vi "Delimiter Write 1.vi"(4 "error in (no error)":errorcluster, 5 "Value":T1, 6 "Container State":T3, 7 "Display State In":T2) -> (0 "error out":errorcluster, 3 "Display State Out":T2)   [LabVIEW 2012, in "Intellisense Xcontrol.xctl"]
uses:
  Intellisense Xcontrol.xctl
  <vilib>/_xctls/Container State.ctl
  State 1.ctl
  Delimiter Enum.ctl
  <vilib>/_xctls/XControlSupport.lvlib
panel:
  # "Replace the Value Control below with a Control of desired type.\nDo not remove this Control or the others from the connector pane.\nDo not change the connector pane pattern.\nThe Value control should always be the third terminal from top on the input side in the connector pane."
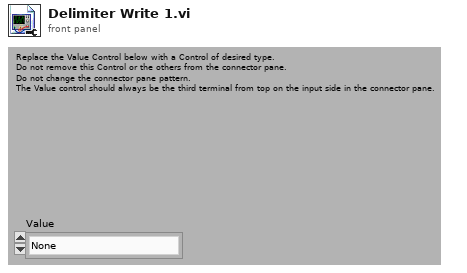
[diagram p1: front panel]
types:
  T1 = typedef "Intellisense Xcontrol.xctl/Delimiter Enum.ctl" = enum16{"None", "Space", "Dash \"-\"", "Slash \"/\"", "Backslash \"\\\"", "Colon", "Period", "Comma", "Line Feed"}
  T2 = typedef "Intellisense Xcontrol.xctl/State 1.ctl" = cluster{"Keyword Array":string[], "Auto-Complete On/Off":bool, "Delimiter":string}
  T3 = typedef "XControlSupport.lvlib/Container State.ctl" = cluster{"Indicator?":bool, "Run Mode?":bool, " Refnum":refnum<vi>}
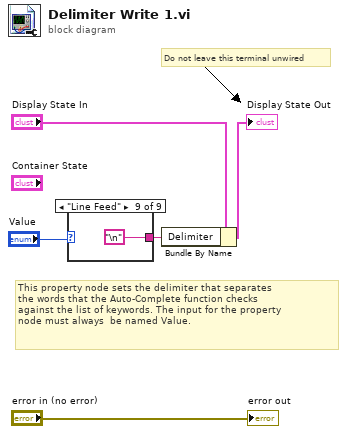
[diagram p0: block diagram]
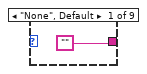
[diagram p2: hidden frame]
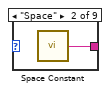
[diagram p3: hidden frame]
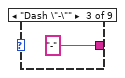
[diagram p4: hidden frame]
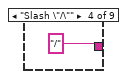
[diagram p5: hidden frame]
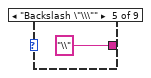
[diagram p6: hidden frame]
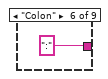
[diagram p7: hidden frame]
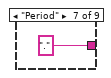
[diagram p8: hidden frame]
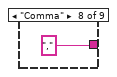
[diagram p9: hidden frame]
diagram:
  # "This property node sets the delimiter that separates\nthe words that the Auto-Complete function checks\nagainst the list of keywords. The input for the property\nnode must always  be named Value."
  # "Do not leave this terminal unwired"
  n1 = case shown="\"Line Feed\"" "Value" {
    tunnel: ["" w7 "-" "/" "\\" ":" "." "," "\n"] -> w1
    frame "None", Default {
    }
    frame "Space" {
      n2 = call <vilib>:"Space Constant.vi"() -> ("String"=w7:string)
    }
    frame "Dash \"-\"" {
    }
    frame "Slash \"/\"" {
    }
    frame "Backslash \"\\\"" {
    }
    frame "Colon" {
    }
    frame "Period" {
    }
    frame "Comma" {
    }
    frame "Line Feed" {
    }
  }
  n3 = Bundle By Name(cluster="Display State In", "Delimiter"=w1) -> (→"Display State Out":T2)
  "error out" <- "error in (no error)"
